vi "uPublisher Register.vi"(6 "uStringManipulation":refnum<class "uStringManipulation.lvclass">, 8 "error in (no error)":errorcluster, 10 "Broker":refnum<class "uTransport_uActor.lvclass">, 11 "Publisher's uTransport":refnum<class "uTransport.lvclass">) -> (0 "error out":errorcluster, 3 "uClient_Publisher out":refnum<class "uClient_Publisher.lvclass">)   [LabVIEW 2023, in "uFramework.lvlib" / "uClient_Publisher.lvclass"]
doc: "Create a publisher client.\nIf a uStringManipulation object is wired in, it is applied to the string when an event is being published."
uses:
  uClient_Publisher.lvclass
  U:/Projects/uFramework/Src/uFramework/uClient/uClient.lvclass
  uTransport_uActor/uTransport_uActor.lvclass
  U:/Projects/uFramework/Src/uFramework/uTransport/uTransport.lvclass
  uTransport/uTransport.lvclass
  Bin/uStringManipulation.lvlibp/uStringManipulation.lvclass
  uMsg/uMsg.lvclass
  uTransport_Queue/uTransport_Queue.lvclass/uTransport_Queue.ctl
  uMsg/uMsg.lvclass/uMsg.ctl
  uClient_Publisher.lvclass/uClient_Publisher.ctl
  uClient/uClient.lvclass/uClient.ctl
  uMsg/uMsg Create.vi
  uMsg/uMsg Get Payload.vi
  uTransport/uTransport_SendMsg.vi
  uTransport_Queue/uTransport_Queue_Create.vi
  uMsg/uMsg Update Timestamp.vi
  uTransport_Queue/uTransport_Queue.lvclass
  <vilib>/Utility/error.llb/Error Cluster From Error Code.vi
  Bin/uData.lvlibp/uData.lvclass
  uClient/uClient.lvclass
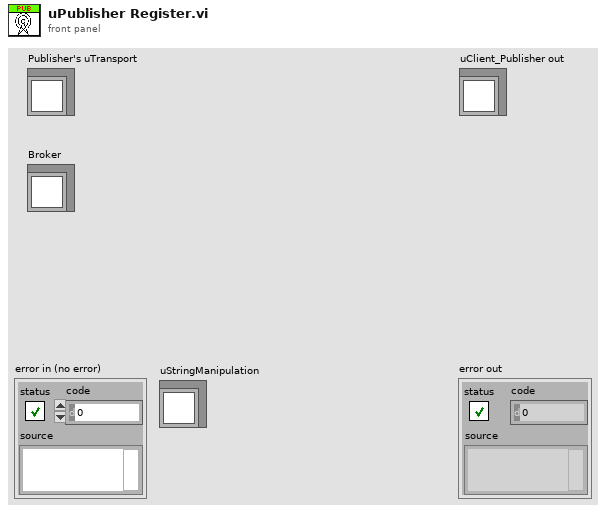
[diagram p1: front panel]
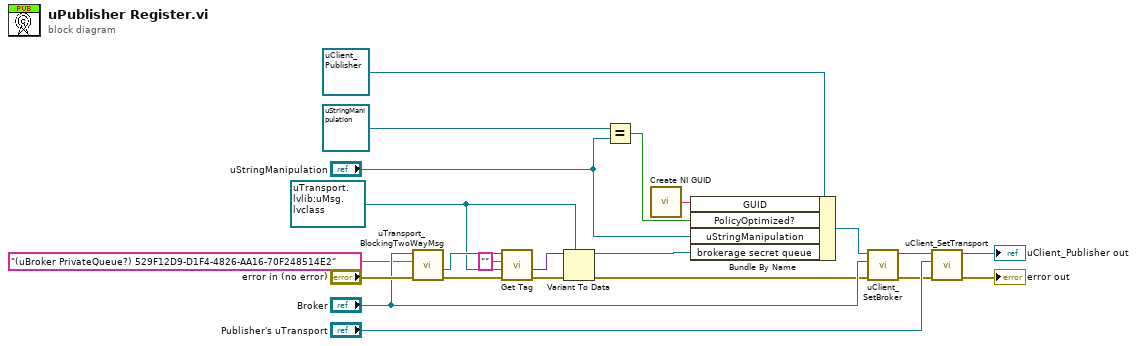
[diagram p0: block diagram]
diagram:
  w5 = refnum<queue> refnum ("brokerage queue")
  n1 = call "uTransport_BlockingTwoWayMsg.vi"("error in (no error)"="error in (no error)", "Command"="(uBroker PrivateQueue?) 529F12D9-D1F4-4826-AA16-70F248514E2", "uTransport in"="Broker") -> ("error out"=w9:errorcluster, "Reply"=w10:refnum<class "uData.lvclass">)  [unwired: 7 in]
  n2 = call "Get Tag.vi"("error in (no error)"=w9, "default value"=w5, "tag (case insensitive)"="", "uData in"=w10) -> ("error out"=w8:errorcluster, "value"=w6:variant)  [unwired: 4 in, 2 out]
  n3 = Variant To Data(error in=w8, type=w5, Variant=w6) -> (data=w11:refnum<queue>, error out=w14:errorcluster)
  n4 = Equal?(x=refnum<class "uStringManipulation.lvclass"> refnum ("uFramework.lvlib:uStringManipulation.lvclass"), y="uStringManipulation") -> (x = y?=w3:bool)
  n5 = call <vilib>:"Create NI GUID.vi"() -> ("NI GUID"=w1:string)
  n6 = Bundle By Name(cluster=refnum<class "uClient_Publisher.lvclass"> refnum ("uClient_Publisher in"), "GUID"=w1, "PolicyOptimized?"=w3, "uStringManipulation"="uStringManipulation", "brokerage secret queue"=w11) -> (w12:refnum<class "uClient_Publisher.lvclass">)
  n7 = call "uClient_SetBroker.vi"("error in (no error)"=w14, "Broker"="Broker", "uClient in"=w12) -> ("error out"=w18:errorcluster, "uClient out"=w19:refnum<class "uClient_Publisher.lvclass">)  [unwired: 7 in]
  n8 = call "uClient_SetTransport.vi"("error in (no error)"=w18, "uTransport"="Publisher's uTransport", "uClient in"=w19) -> ("error out"=→"error out":errorcluster, "uClient out"=→"uClient_Publisher out":refnum<class "uClient_Publisher.lvclass">)  [unwired: 7 in]
